vi "Read Valid Pixels Top Left.vi"(8 "error in (no error)":errorcluster, 11 "Image Undistorter in":refnum<class "Image Undistorter.lvclass">) -> (0 "error out":errorcluster, 2 "Image Point":T1, 3 "Image Undistorter":refnum<class "Image Undistorter.lvclass">)   [LabVIEW 2020, in "image.lvlib" / "Image Undistorter.lvclass"]
doc: "Get the top left corner (origin) of the undistored image valid-pixel region."
uses:
  Image Undistorter.lvclass
  Image Undistorter.lvclass/Image Undistorter.ctl
  common/Image Point (Integer).ctl
  common/common.lvlib
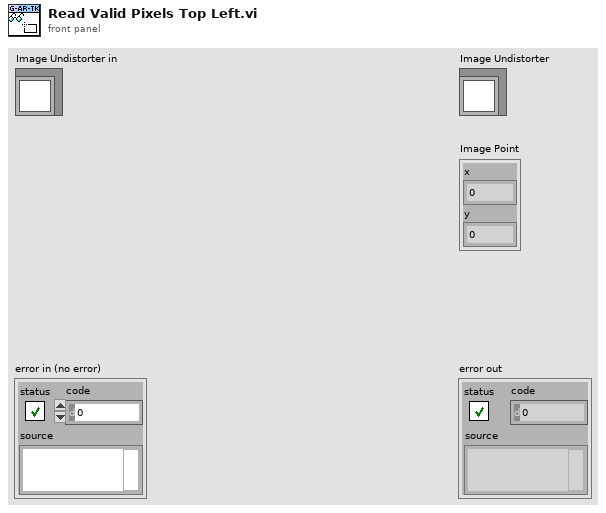
[diagram p1: front panel]
types:
  T1 = typedef "common.lvlib/Image Point (Integer).ctl" = cluster{"x":i32, "y":i32}
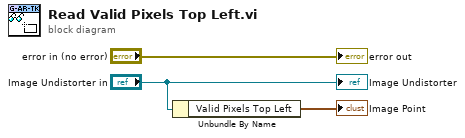
[diagram p0: block diagram]
diagram:
  n1 = Unbundle By Name("Image Undistorter in") -> ("Valid Pixels Top Left"=→"Image Point":T1)
  "error out" <- "error in (no error)"
  "Image Undistorter" <- "Image Undistorter in"
